vi "Connect.vi"(8 "error in (no error)":errorcluster, 9 "Port":u16, 10 "address":string, 11 "RemoteControl in":refnum<class "RemoteControl.lvclass">) -> (0 "error out":errorcluster, 3 "RemoteControl out":refnum<class "RemoteControl.lvclass">)   [LabVIEW 2019, in "RemoteControl.lvclass"]
uses:
  RemoteControl.lvclass
  RemoteControl.lvclass/RemoteControl.ctl
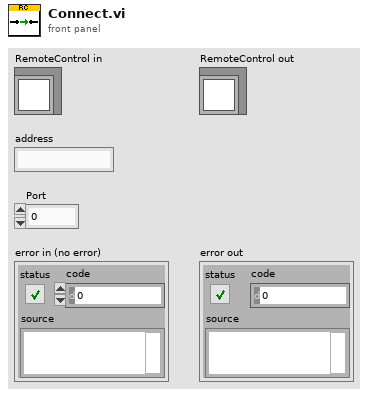
[diagram p1: front panel]
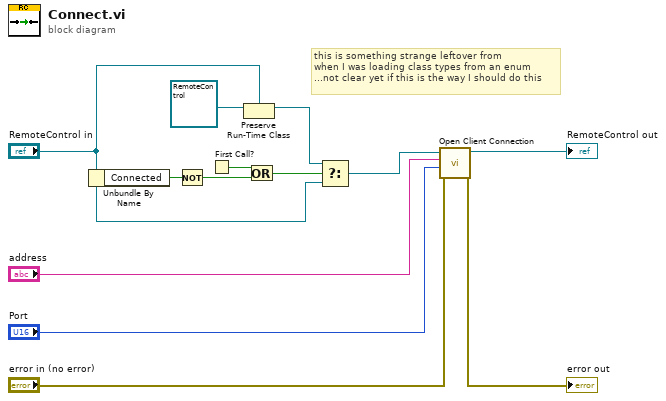
[diagram p0: block diagram]
diagram:
  # "this is something strange leftover from\nwhen I was loading class types from an enum\n...not clear yet if this is the way I should do this"
  n1 = Unbundle By Name("RemoteControl in") -> ("Connected"=w8:bool)
  n2 = Not(x=w8) -> (.not. x?=w7:bool)
  n3 = First Call?() -> (First Call?: T/F=w9:bool)
  n4 = Preserve Run-Time Class(object in=refnum<class "RemoteControl.lvclass"> refnum ("RemoteControl in"), 2:"RemoteControl in") -> (object out=w3:refnum<class "RemoteControl.lvclass">)  [unwired: 1 in, 1 out]
  n5 = Or(x=w9, y=w7) -> (x .or. y?=w6:bool)
  n6 = Select(t=w3, s=w6, f="RemoteControl in") -> (s? t:f=w1:refnum<class "RemoteControl.lvclass">)
  n7 = call-dynamic "Open Client Connection.vi"("error in (no error)"="error in (no error)", "Port"="Port", "address"="address", "RemoteControl in"=w1) -> ("error out"=→"error out":errorcluster, "RemoteControl out"=→"RemoteControl out":refnum<class "RemoteControl.lvclass">)  [unwired: 6 in]
